vi "S2C_ExeBreakOnFail.vi"(8 "Error In":errorcluster, 10 "LastStep?":bool, 11 "Q_Ref":refnum<queue>) -> (0 "Error Out":errorcluster, 3 "IncRow?":bool)   [LabVIEW 2015]
uses:
  Controls/S2C_ExePause.ctl
  Globals/S2C_Globals.vi
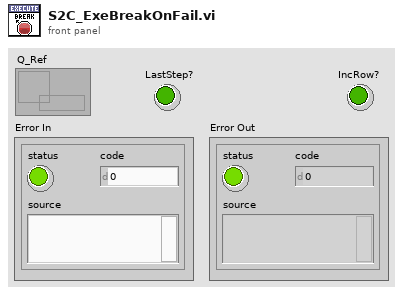
[diagram p1: front panel]
types:
  T1 = typedef "S2C_ExePause.ctl" = bool
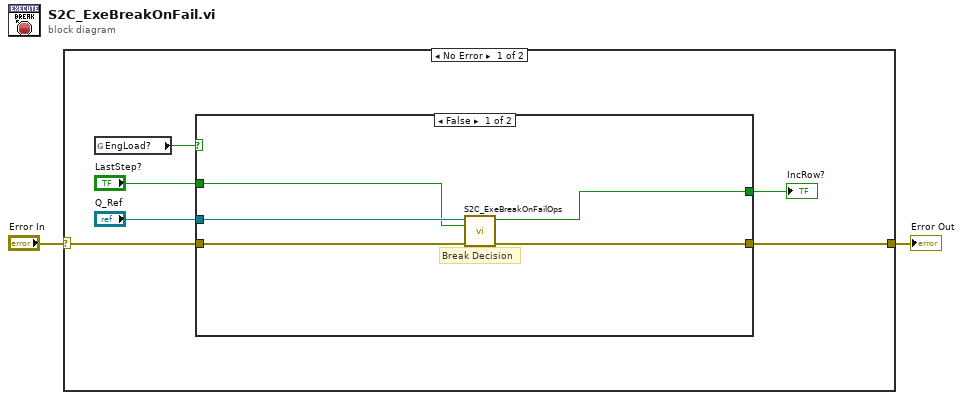
[diagram p0: block diagram]
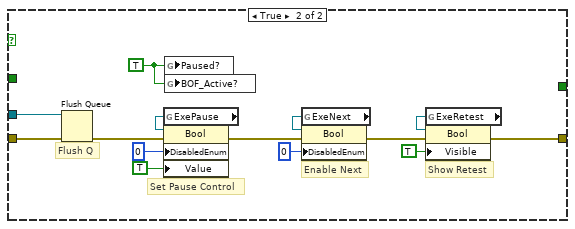
[diagram p2: hidden frame]
diagram:
  n1 = case shown="No Error" "Error In" {
    selector: "Error In" -> [w8 w28]
    tunnel: [w7 w28] -> w1
    frame No Error {
      n2 = global read "S2C_Globals.vi" "EngLoad?"() -> (w6:bool)
      n3 = case shown="False" w6 {
        tunnel: w8 -> [w13 w21]
        tunnel: [w11 w14] -> w7
        tunnel: "Q_Ref" -> [w12 w19]
        tunnel: [w10 _] -> w4
        tunnel: "LastStep?" -> [w9 _]
        frame False {
          # "Break Decision"
          n4 = call "S2C_ExeBreakOnFailOps.vi"("Error In"=w13, "LastStep?"=w9, "Q_Ref"=w12) -> ("Error Out"=w11:errorcluster, "IncRow?"=w10:bool)  [unwired: 7 in]
        }
        frame True {
          w18 = TRUE ("Paused?")
          # "Show Retest"
          # "Flush Q"
          # "Set Pause Control"
          # "Enable Next"
          n5 = Flush Queue(queue=w19, error in (no error)=w21) -> (error out=w20:errorcluster)  [unwired: 2 out]
          n6 = global read "S2C_Globals.vi" "ExePause"() -> (w25:refnum<vi>)
          n7 = property on="Property Node" class="Bool"(reference=w25, error in=w20, "DisabledEnum"=u8 0, "Value"=T1 TRUE) -> (error out=w24:errorcluster)  [unwired: 1 out]
          n8 = global write "S2C_Globals.vi" "Paused?"(w18) -> ()
          n9 = global write "S2C_Globals.vi" "BOF_Active?"(w18) -> ()
          n10 = global read "S2C_Globals.vi" "ExeNext"() -> (w27:refnum<vi>)
          n11 = property on="Property Node" class="Bool"(reference=w27, error in=w24, "DisabledEnum"=u8 0) -> (error out=w16:errorcluster)  [unwired: 1 out]
          n12 = global read "S2C_Globals.vi" "ExeRetest"() -> (w17:refnum<vi>)
          n13 = property on="Property Node" class="Bool"(reference=w17, error in=w16, "Visible"=TRUE) -> (error out=w14:errorcluster)  [unwired: 1 out]
        }
      }
      "IncRow?" <- w4
    }
    frame Error {
    }
  }
  "Error Out" <- w1
